vi "Test.vi"() -> ()   [LabVIEW 2016, in "Stepper Motor Controller.lvlib" / "KST101.lvclass"]
uses:
  KST101.lvclass
  TypeDefs/KST-MotorSettings.ctl
  TypeDefs/KST-HomeConfig.ctl
  TypeDefs/KST-JogConfig.ctl
  KST101.lvclass/KST101.ctl
panel:
  in  "serialNumber":string="26001631"
  out "currentPosition":dbl
  out "configError":errorcluster
  out "error out":errorcluster
  in  "Home Button":bool
  in  "jogDistance":dbl=0.1
  in  "moveDestination":dbl
  in  "Jog Button":bool
  in  "Move Button":bool
  in  "Stop Button":bool
  in  "motorSettings":T1={"maxVelocity"=1.0, "acceleration"=0.5, "maxTravel"=0.0, "minTravel"=0.0, "waitTimeout"=60000, "stageType"=50, "units"="", "homeConfig"={"direction"=2, "limitSwitch"=1, "offsetDistance"=0.1, "velocity"=0.5, "waitTimeout"=60000, "postHomeTravel"=0.0}, "jogSettings"={"jogSize"=0.1, "maxVelocity"=1.0, "acceleration"=0.5, "waitTimeout"=60000}, "Setup Offset"=0.0} {"stageType" items=["ZST6"=32, "ZST13"=33, "ZST25"=34, "ZST206"=48, "ZST213"=49, "ZST225"=50, "ZFS206"=64, "ZFS213"=65, "ZFS225"=66, "NR360"=112, "PLS_X25MM"=114, "PLS_X25MM_HiRes"=115, "FW103"=117]; "homeConfig"."limitSwitch" items=["Ignore"=0, "ClockwiseHard"=1, "CounterClockwiseHard"=4]; "homeConfig"."direction" items=["Clockwise"=1, "CounterClockwise"=2]}
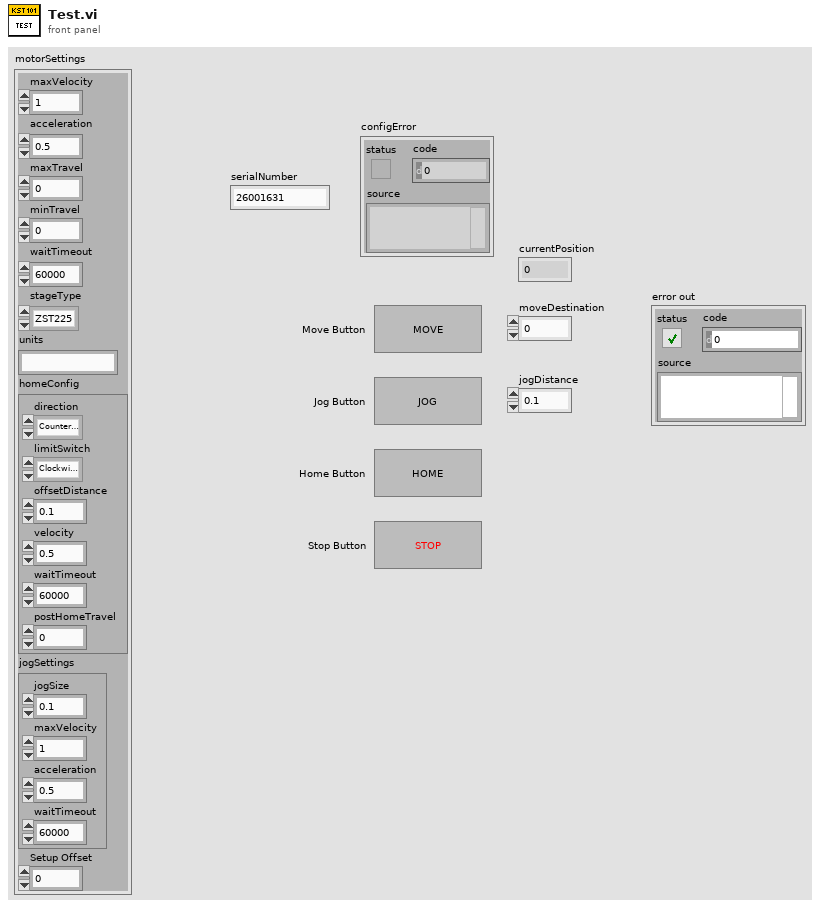
[diagram p1: front panel]
types:
  T1 = typedef "Stepper Motor Controller.lvlib/KST101.lvclass/KST-MotorSettings.ctl" = cluster{"maxVelocity":dbl, "acceleration":dbl, "maxTravel":dbl, "minTravel":dbl, "waitTimeout":i32, "stageType":i32, "units":string, "homeConfig":T2, "jogSettings":T3, "Setup Offset":dbl}
  T2 = typedef "Stepper Motor Controller.lvlib/KST101.lvclass/KST-HomeConfig.ctl" = cluster{"direction":i32, "limitSwitch":i32, "offsetDistance":dbl, "velocity":dbl, "waitTimeout":i32, "postHomeTravel":dbl}
  T3 = typedef "Stepper Motor Controller.lvlib/KST101.lvclass/KST-JogConfig.ctl" = cluster{"jogSize":dbl, "maxVelocity":dbl, "acceleration":dbl, "waitTimeout":i32}
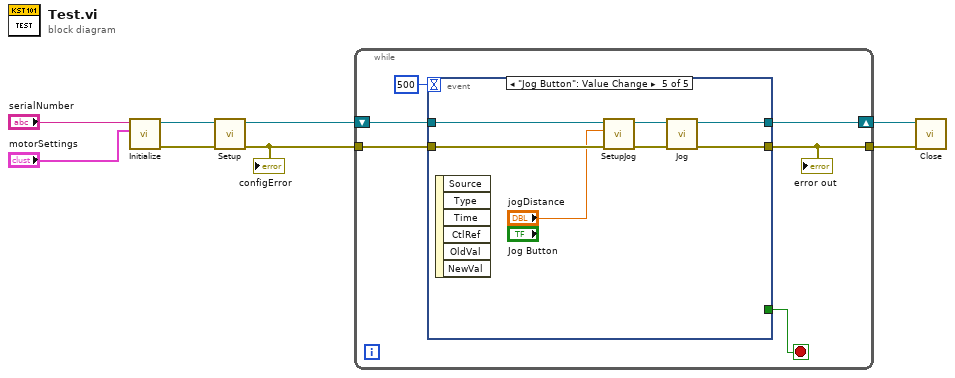
[diagram p0: block diagram]
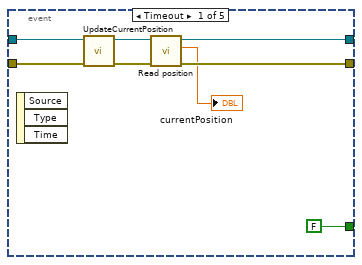
[diagram p2: hidden frame]
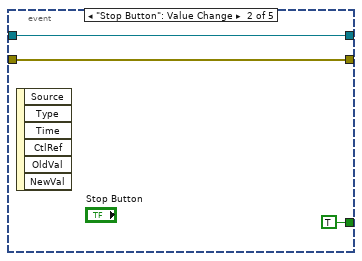
[diagram p3: hidden frame]
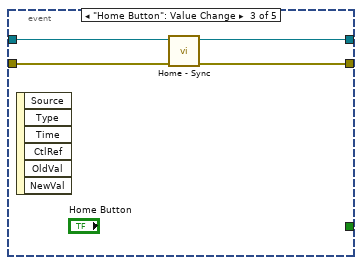
[diagram p4: hidden frame]
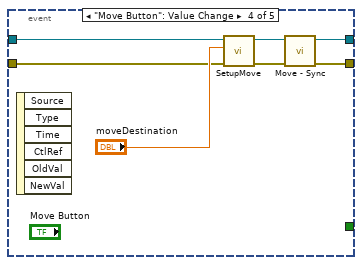
[diagram p5: hidden frame]
diagram:
  n1 = call "Initialize.vi"("motorSettings"="motorSettings", "serialNumber"="serialNumber") -> ("error out"=w7:errorcluster, "KST101 out"=w8:refnum<class "KST101.lvclass">)  [unwired: 8 in]
  n2 = call-dynamic "Setup.vi"("error in (no error)"=w7, "KST101 in"=w8) -> ("error out"=w3:errorcluster, "KST101 out"=w4:refnum<class "KST101.lvclass">)  [unwired: 8 in]
  "configError" <- w3
  n3 = while {
    shift-right: [w11] -> w2
    shift-left: w4 -> [w14]
    tunnel: w3 -> [w12]
    tunnel: [w10] -> w1
    stop <- w9 stop-if-true
    n4 = event shown="[4] \"Jog Button\": Value Change" {
      selector: _ -> [_ _ _ _ _]
      dyn-events: _ -> [_ _ _ _ _]
      timeout: 500 -> [_ _ _ _ _]
      tunnel: w14 -> [w20 w25 w29 w34 w42]
      tunnel: w12 -> [w17 w24 w27 w31 w39]
      tunnel: [w19 w25 w28 w33 w41] -> w11
      tunnel: [w16 w24 w26 w30 w38] -> w10
      tunnel: [FALSE TRUE _ _ _] -> w9
      event Timeout {
        n5 = event-data() -> ()  [unwired: 1 in, 3 out]
        n6 = call-dynamic "UpdateCurrentPosition.vi"("error in (no error)"=w17, "KST101 in"=w20) -> ("error out"=w18:errorcluster, "KST101 out"=w21:refnum<class "KST101.lvclass">)  [unwired: 8 in]
        n7 = call "Read position.vi"("error in (no error)"=w18, "KST101 in"=w21) -> ("error out"=w16:errorcluster, "position"=→"currentPosition":dbl, "KST101 out"=w19:refnum<class "KST101.lvclass">)  [unwired: 7 in]
      }
      event "Stop Button": Value Change {
        n8 = event-data() -> ()  [unwired: 1 in, 6 out]
      }
      event "Home Button": Value Change {
        n9 = event-data() -> ()  [unwired: 1 in, 6 out]
        n10 = call-dynamic "Home - Sync.vi"("error in (no error)"=w27, "KST101 in"=w29) -> ("error out"=w26:errorcluster, "KST101 out"=w28:refnum<class "KST101.lvclass">)  [unwired: 8 in]
      }
      event "Move Button": Value Change {
        n11 = event-data() -> ()  [unwired: 1 in, 6 out]
        n12 = call-dynamic "SetupMove.vi"("error in (no error)"=w31, "moveDestination"="moveDestination", "KST101 in"=w34) -> ("error out"=w32:errorcluster, "KST101 out"=w35:refnum<class "KST101.lvclass">)  [unwired: 7 in]
        n13 = call-dynamic "Move - Sync.vi"("error in (no error)"=w32, "KST101 in"=w35) -> ("error out"=w30:errorcluster, "KST101 out"=w33:refnum<class "KST101.lvclass">)  [unwired: 8 in]
      }
      event "Jog Button": Value Change {
        n14 = event-data() -> ()  [unwired: 1 in, 6 out]
        n15 = call-dynamic "SetupJog.vi"("error in (no error)"=w39, "jogDistance"="jogDistance", "KST101 in"=w42) -> ("error out"=w40:errorcluster, "KST101 out"=w43:refnum<class "KST101.lvclass">)  [unwired: 7 in]
        n16 = call-dynamic "Jog.vi"("error in (no error)"=w40, "KST101 in"=w43) -> ("error out"=w38:errorcluster, "KST101 out"=w41:refnum<class "KST101.lvclass">)  [unwired: 8 in]
      }
    }
    "error out" <- w10
  }
  n17 = call-dynamic "Close.vi"("error in (no error)"=w1, "KST101 in"=w2) -> ()  [unwired: 9 in, 1 out]
